vi "APS relative helix move.vi"(0 "Dimension":i32, 1 "Pitch":i32, 2 "CwOrCcw":i32, 5 "Axis_ID_Array":i32, 7 "Center_PosOffset_Array":i32, 9 "Max_Arc_Speed":i32, 11 "error in (no error)":errorcluster caption="错误输入（无错误）", 12 "TotalHeight":i32) -> (4 "function return":i32, 6 "Axis_ID_Array out":i32, 8 "Center_PosOffset_Array out":i32, 15 "error out":errorcluster caption="错误输出")   [LabVIEW 2011, in "APS168.lvlib"]
doc: "I32 FNTYPE APS_relative_helix_move( I32 Dimension, I32 *Axis_ID_Array, I32 *Center_PosOffset_Array, I32 Max_Arc_Speed, I32 Pitch, I32 TotalHeight, I32 CwOrCcw );"
uses:
  APS168.lvlib
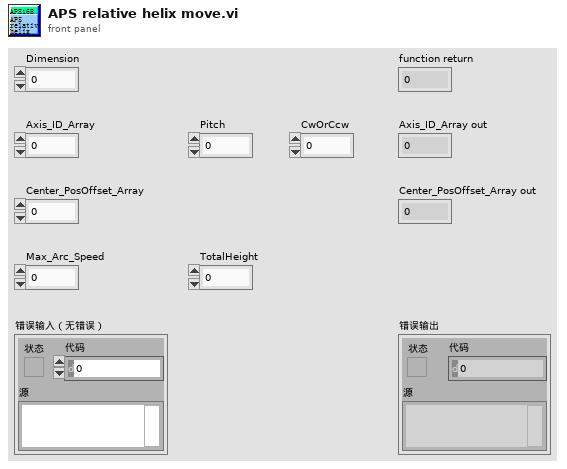
[diagram p1: front panel]
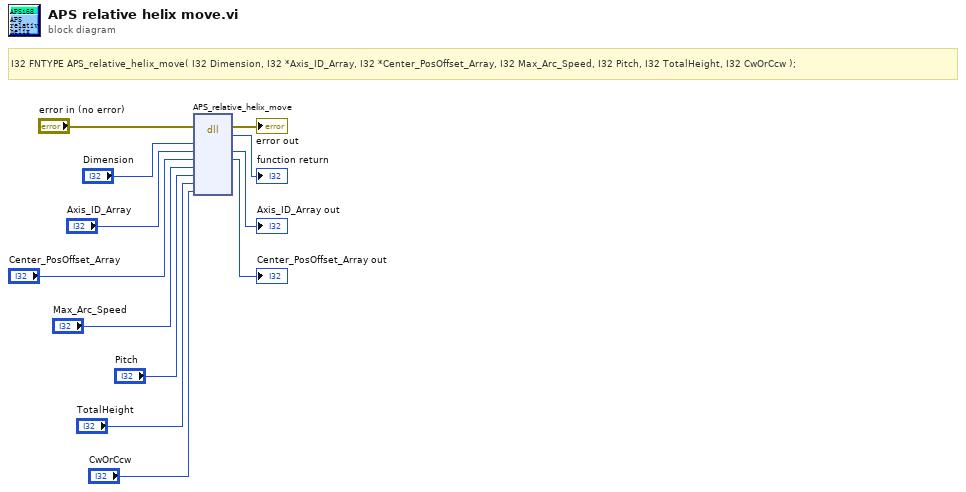
[diagram p0: block diagram]
diagram:
  # "I32 FNTYPE APS_relative_helix_move( I32 Dimension, I32 *Axis_ID_Array, I32 *Center_PosOffset_Array, I32 Max_Arc_Speed, I32 Pitch, I32 TotalHeight, I32 CwOrCcw );"
  n1 = dll-call lib="PTH1Labs E软件ADLINK 204CAPS_1_7_1_LIB line 连续运动204APS168.*" fn="APS_relative_helix_move"(error in="error in (no error)", "Dimension"="Dimension", "Axis_ID_Array"="Axis_ID_Array", "Center_PosOffset_Array"="Center_PosOffset_Array", "Max_Arc_Speed"="Max_Arc_Speed", "Pitch"="Pitch", "TotalHeight"="TotalHeight", "CwOrCcw"="CwOrCcw") -> (error out=→"error out":errorcluster, →"function return":i32, "Axis_ID_Array"=→"Axis_ID_Array out":i32, "Center_PosOffset_Array"=→"Center_PosOffset_Array out":i32)  [unwired: 7 in, 1 out]
